vi "Release Queues.vi"(8 "error in":errorcluster) -> (0 "error out":errorcluster)   [LabVIEW 2019]
doc: "Release all queues.\n\n-----\nJuan Navarro\nLab it Studio"
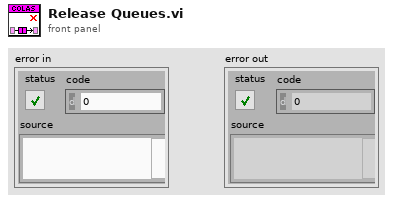
[diagram p1: front panel]
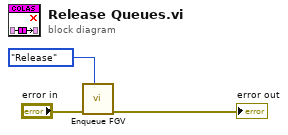
[diagram p0: block diagram]
diagram:
  n1 = call "Enqueue FGV.vi"("Actions"=enum16{"Release", "Flush", "Enqueue", "Get Ref"}."Release", "error in"="error in") -> ("error out"=→"error out":errorcluster)  [unwired: 8 in, 1 out]
